vi "Clear Scalar Channels.vi"(8 "error in":errorcluster, 11 "FPGA Addon refnum in":T1=18446744073709551615 format="%.0x") -> (0 "error out":errorcluster, 3 "FPGA Addon refnum out":T1=18446744073709551615 format="%.0x")   [LabVIEW 2019, in "Scripting API.lvlib"]
uses:
  Scripting API.lvlib
  <vilib>/NI VeriStand/Custom Device API/Custom Device Item Ref.ctl
  Addon/Addon Shared/SubVIs/Constants.vi
  <vilib>/NI/NI VeriStand Advanced SysDef API/_SubVIs/SysDef.Search.GUID.vi
  Addon/Addon Shared/FPGA Addon Shared.lvlib
  <vilib>/NI/NI VeriStand Advanced SysDef API/SysDef API/Advanced System Definition.lvlib
  <vilib>/NI VeriStand/Custom Device API/Custom Device API.lvlib
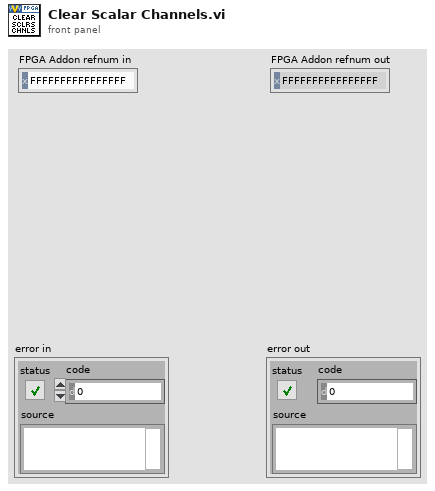
[diagram p1: front panel]
types:
  T1 = typedef "Custom Device API.lvlib/Custom Device Item Ref.ctl" = u64
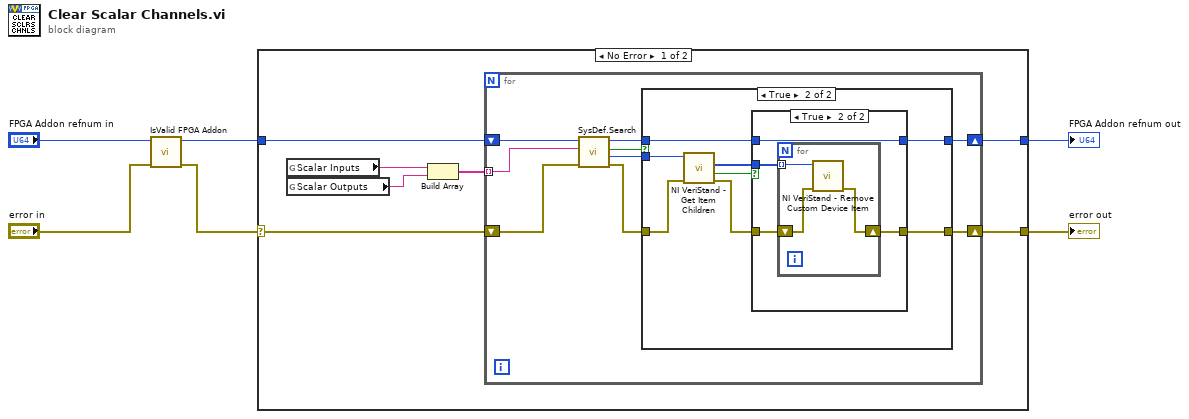
[diagram p0: block diagram]
diagram:
  n1 = call "IsValid FPGA Addon.vi"("error in"="error in", "FPGA Addon refnum in"="FPGA Addon refnum in") -> ("error out"=w1:errorcluster, "FPGA Addon refnum out"=w3:T1)  [unwired: 8 in]
  n2 = case shown="No Error" w1 {
    selector: w1 -> [w9 w42]
    tunnel: w3 -> [w11 w43]
    tunnel: [w8 w43] -> w6
    tunnel: [w7 w42] -> w5
    frame No Error {
      n3 = global read "Constants.vi" "Scalar Inputs"() -> (w13:string)
      n4 = global read "Constants.vi" "Scalar Outputs"() -> (w12:string)
      n5 = Build Array(w13, w12) -> (w10:string[])
      n6 = for {
        tunnel: w10 -> [w22] mode=indexing
        shift-right: [w16] -> w8
        shift-left: w11 -> [w21]
        shift-right: [w14] -> w7
        shift-left: w9 -> [w19]
        n7 = call-poly <vilib>:"SysDef.Search.vi"("error in (no error)"=w19, "GUID"=w22, "nodeID"=w21) -> ("error out"=w18:errorcluster, "Value out"=w20:u64, "nodeID out"=w17:u64, "Found?"=w15:bool)  [unwired: 5 in]
        n8 = case shown="True" w15 {
          tunnel: w20 -> [_ w32]
          tunnel: w18 -> [w23 w30]
          tunnel: w17 -> [w24 w27]
          tunnel: [w24 w26] -> w16
          tunnel: [w23 w25] -> w14
          frame False {
          }
          frame True {
            n9 = call <vilib>:"NI VeriStand - Get Item Children.vi"("error in (no error)"=w30, "Item Ref in"=w32) -> ("error out"=w29:errorcluster, "Child Refs"=w31:T1[], "Found"=w28:bool)  [unwired: 6 in, 1 out]
            n10 = case shown="True" w28 {
              tunnel: w31 -> [_ w38]
              tunnel: w29 -> [w33 w37]
              tunnel: w27 -> [w34 w36]
              tunnel: [w34 w36] -> w26
              tunnel: [w33 w35] -> w25
              frame False {
              }
              frame True {
                n11 = for {
                  tunnel: w38 -> [w41] mode=indexing
                  shift-right: [w39] -> w35
                  shift-left: w37 -> [w40]
                  n12 = call <vilib>:"NI VeriStand - Remove Custom Device Item.vi"("error in (no error)"=w40, "Item Ref in"=w41) -> ("error out"=w39:errorcluster)  [unwired: 8 in, 1 out]
                }
              }
            }
          }
        }
      }
    }
    frame Error {
    }
  }
  "error out" <- w5
  "FPGA Addon refnum out" <- w6
